vi "GFGallGet.vi"(7 "GFG Refnum (use when calling from external project)":refnum<vi>, 8 "error in (no error)":errorcluster) -> (0 "error out":errorcluster, 3 "Array of Clusters of Variables":T2(array[cluster]))   [LabVIEW 2012, in "GFG library.lvlib"]
uses:
  GFG library.lvlib
  <vilib>/Utility/VariantDataType/Type.ctl
  <vilib>/Utility/VariantDataType/VariantType.lvlib
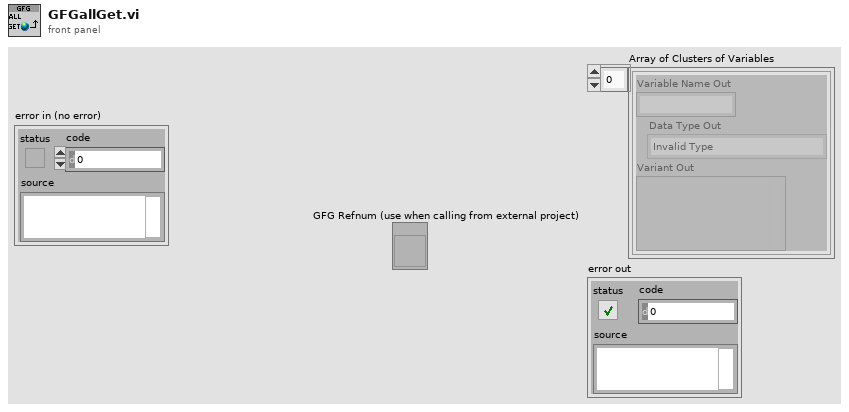
[diagram p1: front panel]
types:
  T1 = typedef "VariantType.lvlib/Type.ctl" = enum8{"Invalid Type", "Void", "I8", "I16", "I32", "I64", "U8", "U16", "U32", "U64", "Single Float", "Double Float", "Extended Float", "Single Complex", "Double Complex", "Extended Complex", "Enum U8", "Enum U16", "Enum U32", "Enum U64", "Single Float With Unit", "Double Float With Unit", "Extended Float With Unit", "Single Complex with Unit", "Double Complex with Unit", "Extended Complex with Unit", "Boolean", "String", "Path", "Picture", "Tag", "Array", "Cluster", "Variant", "LV Variant", "Waveform", "Timestamp", "Digital Waveform", "Digital Data", "ExpressData", "Refnum", "External Data", "VI", "Poly VI", "LabVIEW Class Instance", "Fixed Point"}
  T2 = cluster{"Variable Name Out":string, "Data Type Out":T1, "Variant Out":variant}[]
  T3 = cluster{"Variable Name Out":string, "Data Type Out":T1, "Variant Out":variant}
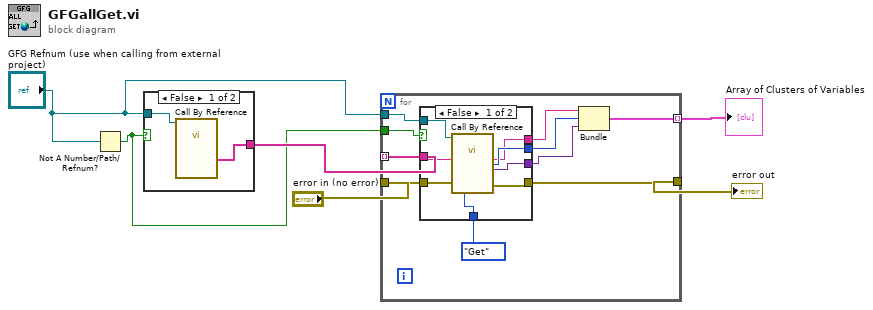
[diagram p0: block diagram]
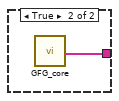
[diagram p2: hidden frame]
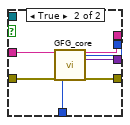
[diagram p3: hidden frame]
diagram:
  n1 = Not A Number/Path/Refnum?(number/path/refnum="GFG Refnum (use when calling from external project)") -> (NaN/Path/Refnum?=w2:bool)
  n2 = case shown="False" w2 {
    tunnel: [w7 w9] -> w4
    tunnel: "GFG Refnum (use when calling from external project)" -> [w8 _]
    frame False {
      n3 = call-by-ref "?"(reference=w8) -> ("All Variable Names Out"=w7:string[])  [unwired: 14 in, 8 out]
    }
    frame True {
      n4 = call "GFG_core.vi"() -> ("All Variable Names Out"=w9:string[])  [unwired: 13 in, 6 out]
    }
  }
  n5 = for {
    tunnel: w4 -> [w18] mode=indexing
    tunnel: "error in (no error)" -> [w17]
    tunnel: [w16] -> w5
    tunnel: [w12] -> w6 mode=indexing
    tunnel: w2 -> [w11]
    tunnel: "GFG Refnum (use when calling from external project)" -> [w10]
    n6 = case shown="False" w11 {
      tunnel: enum16{"Init", "Set", "Get"}."Get" ("Action") -> [w21 w34]
      tunnel: w18 -> [w22 w33]
      tunnel: w17 -> [w27 w32]
      tunnel: [w26 w31] -> w16
      tunnel: [w23 w30] -> w15
      tunnel: [w24 w29] -> w14
      tunnel: [w25 w28] -> w13
      tunnel: w10 -> [w20 _]
      frame False {
        n7 = call-by-ref "?"(reference=w20, "Variable Name in"=w22, "error in (no error)"=w27, "Action"=w21) -> ("Variable Name Out"=w23:string, "Data Type Out"=w24:T1, "Variant Out"=w25:variant, "error out"=w26:errorcluster)  [unwired: 11 in, 5 out]
      }
      frame True {
        n8 = call "GFG_core.vi"("Variable Name in"=w33, "error in (no error)"=w32, "Action"=w34) -> ("Variable Name Out"=w30:string, "Data Type Out"=w29:T1, "Variant Out"=w28:variant, "error out"=w31:errorcluster)  [unwired: 10 in, 3 out]
      }
    }
    n9 = Bundle("Variable Name Out"=w15, "Data Type Out"=w14, "Variant Out"=w13) -> (w12:T3)  [unwired: 1 in]
  }
  "error out" <- w5
  "Array of Clusters of Variables" <- w6
